vi "MFCSetpoint.vi"(8 "MFC error in":errorcluster, 10 "MFC setpoint":dbl, 11 "MFC VISA in":refnum<visa-resource-name>) -> (0 "MFC error out":errorcluster, 3 "MFC VISA out":refnum<visa-resource-name>)   [LabVIEW 2018]
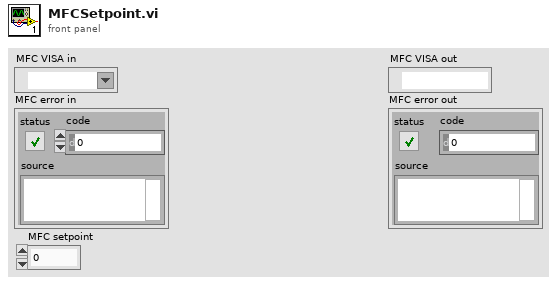
[diagram p1: front panel]
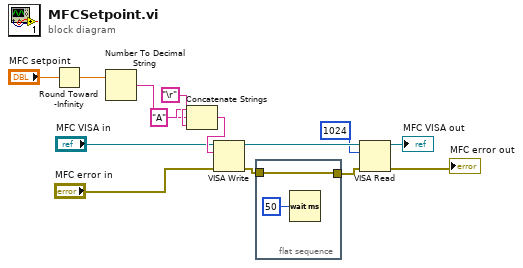
[diagram p0: block diagram]
diagram:
  n1 = Round Toward -Infinity(1:"MFC setpoint") -> (0:w2:dbl)
  n2 = Number To Decimal String(number=w2) -> (decimal integer string=w3:string)  [unwired: 1 in]
  n3 = Concatenate Strings("A" ("write buffer"), w3, "\r") -> (w14:string)
  n4 = VISA Write(VISA resource name="MFC VISA in", write buffer=w14, error in (no error)="MFC error in") -> (VISA resource name out=w12:refnum<visa-resource-name>, error out=w10:errorcluster)  [unwired: 1 out]
  n5 = flat-sequence {
    tunnel: w10 -> [w16]
    tunnel: [w16] -> w9
    frame #0 {
      n6 = Wait (ms)(milliseconds to wait=u32 50) -> ()  [unwired: 1 out]
    }
  }
  n7 = VISA Read(VISA resource name=w12, byte count=u32 1024, error in (no error)=w9) -> (VISA resource name out=→"MFC VISA out":refnum<visa-resource-name>, error out=→"MFC error out":errorcluster)  [unwired: 2 out]
